vi "TempControl.vi"(0 "Param":sgl[](array[numeric])=[0.0, 0.0, 0.0, 0.0, 100.0, 10.0, 0.01, 0.005]) -> ()   [LabVIEW 2015]
uses:
  <vilib>/Instr/_visa.llb/VISA Configure Serial Port (Instr).vi
panel:
  out "error out 5":errorcluster
  in  "error in (no error) 5":errorcluster
  out "error out 4":errorcluster
  in  "error in (no error) 4":errorcluster
  out "error out 3":errorcluster
  in  "error in (no error) 3":errorcluster
  out "error out 2":errorcluster
  in  "error in (no error) 2":errorcluster
  in  "error in (no error)":errorcluster
  out "error out":errorcluster
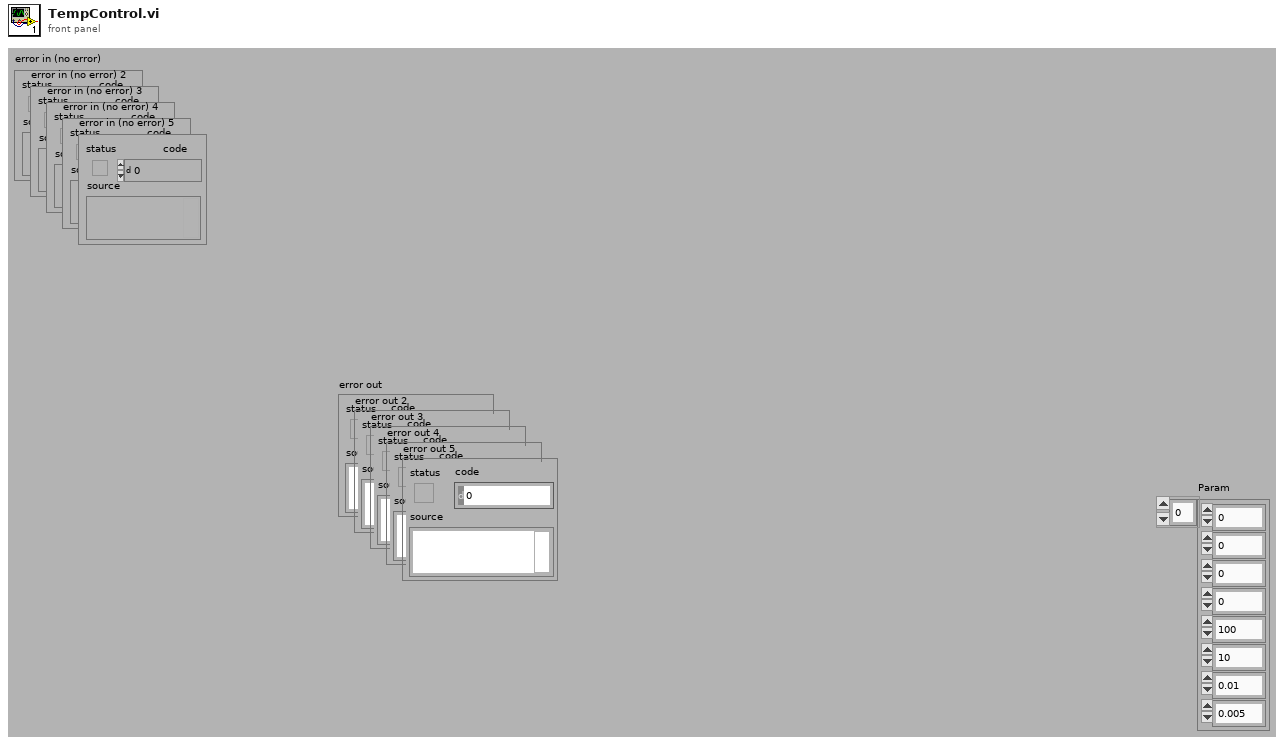
[diagram p1: front panel]
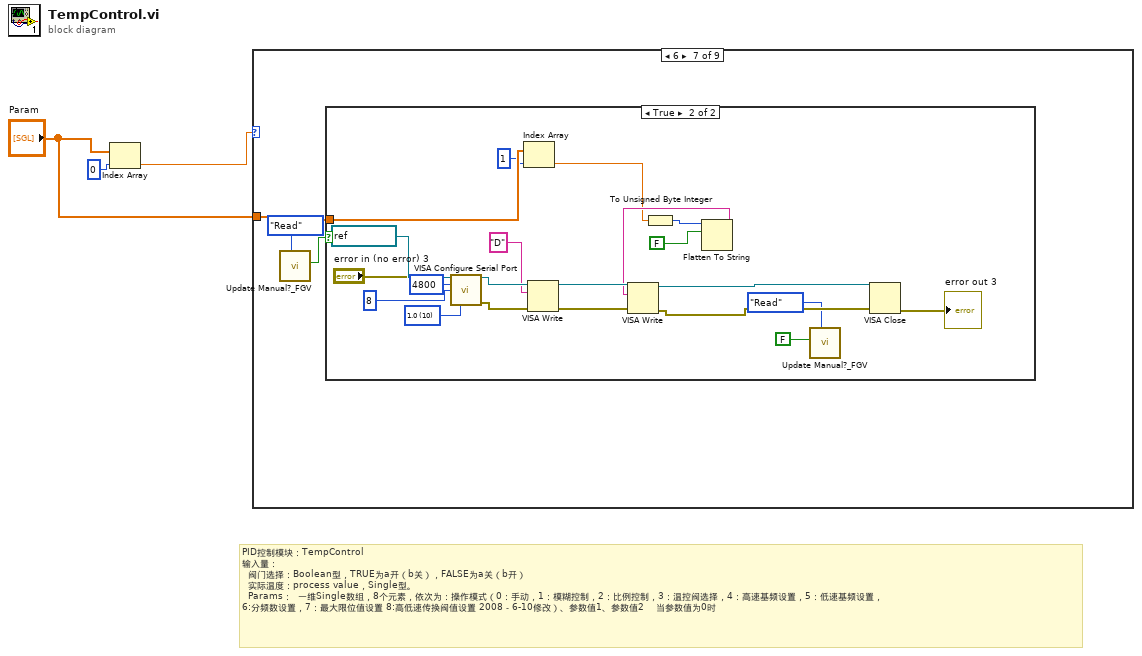
[diagram p0: block diagram]
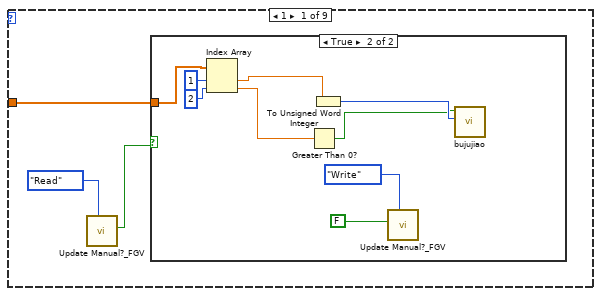
[diagram p2: hidden frame]
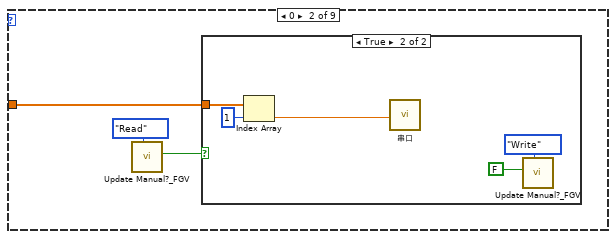
[diagram p4: hidden frame]
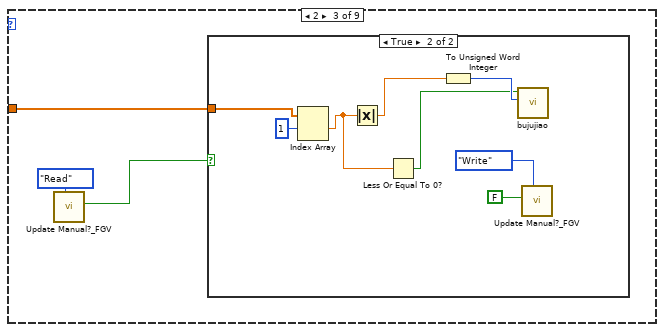
[diagram p6: hidden frame]
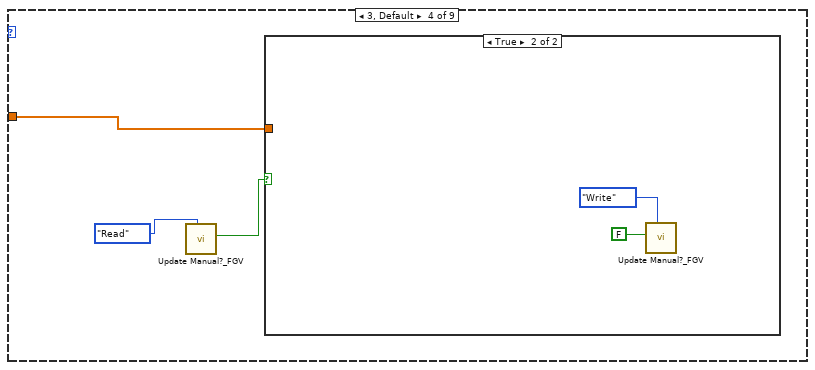
[diagram p8: hidden frame]
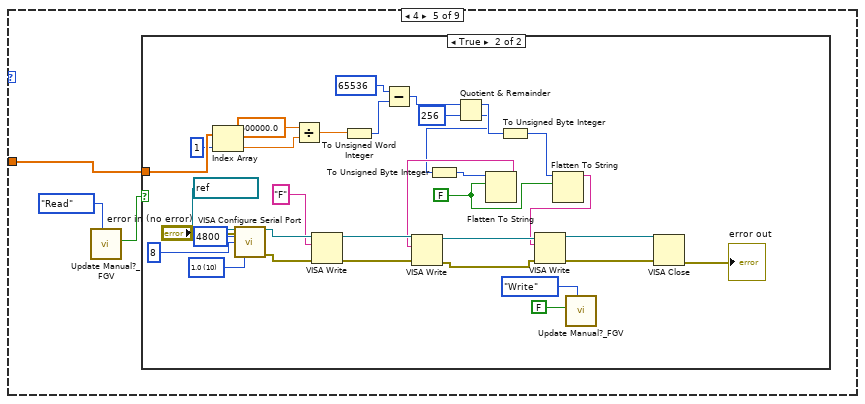
[diagram p10: hidden frame]
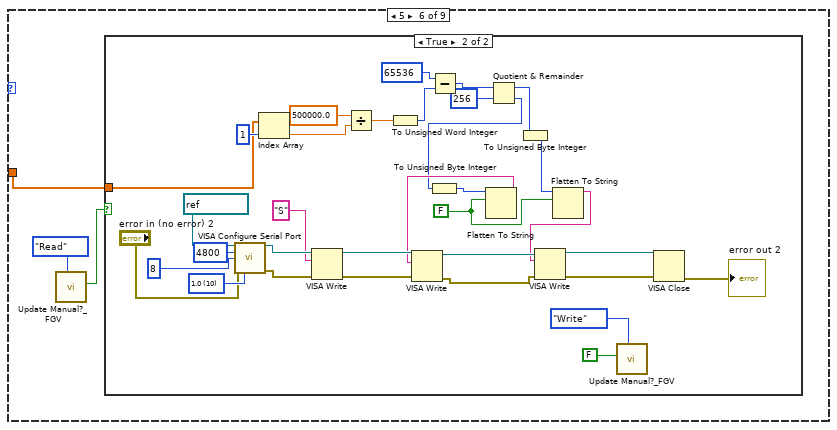
[diagram p12: hidden frame]
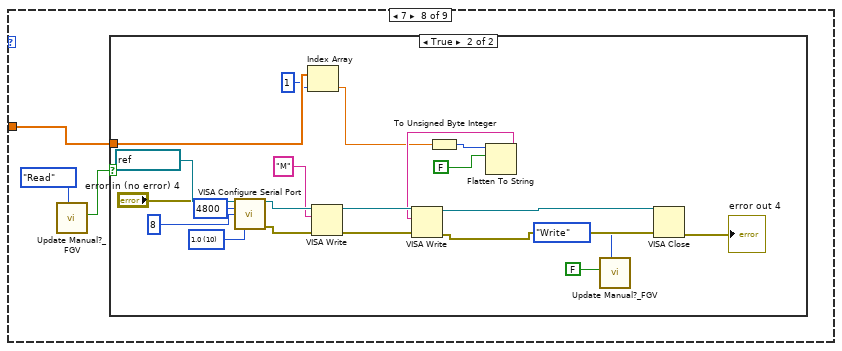
[diagram p15: hidden frame]
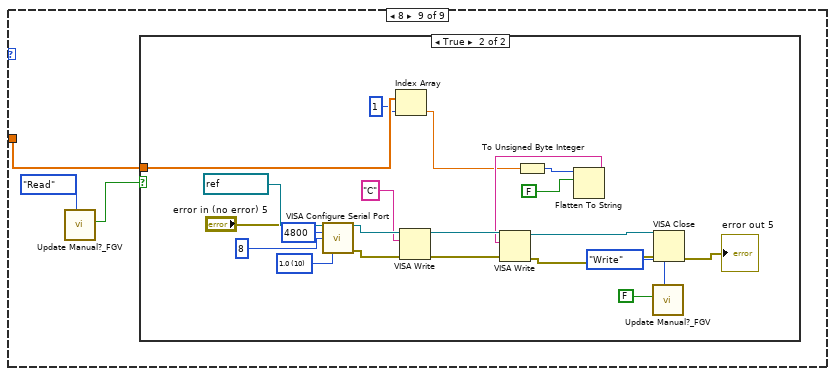
[diagram p17: hidden frame]
diagram:
  # "PID控制模块：TempControl\n输入量： \n \t阀门选择：Boolean型，TRUE为a开（b关），FALSE为a关（b开）\n \t实际温度：process value，Single型。\n \tParams：  一维Single数组，8个元素，依次为：操作模式（0：手动，1：模糊控制，2：比例控制，3：温控阀选择，4：高速基频设置，5：低速基频设置，\n6:分频数设置，7：最大限位值设置 8:高低速传换阀值设置 2008－6-10修改）、参数值1、参数值2    当参数值为0时"
  n1 = Index Array(array="Param", index=0) -> (element=w2:sgl)
  n2 = case shown="6" w2 {
    tunnel: "Param" -> [w6 w18 w26 w35 w42 w78 w114 w138 w162]
    frame 1 {
      n3 = call "Update Manual?_FGV.vi"("W/R"=enum16{"Write", "Read"}."Read") -> ("Update Manual Output?"=w4:bool)  [unwired: 10 in]
      n4 = case shown="True" w4 {
        tunnel: w6 -> [_ w15]
        frame False {
        }
        frame True {
          n5 = Index Array(array=w15, index #1=1 ("index"), index #2=2 ("index")) -> (element #1=w13:sgl, element #2=w10:sgl)
          n6 = Greater Than 0?(x=w10) -> (x > 0?=w9:bool)
          n7 = To Unsigned Word Integer(number=w13) -> (unsigned 16bit integer=w11:u16)
          n8 = call "Update Manual?_FGV.vi"("W/R"=enum16{"Write", "Read"}."Write", "Update Manual?"=FALSE) -> ()  [unwired: 9 in, 1 out]
          n9 = call "bujujiao.vi"("stepnum"=w11, "OK Button"=w9) -> ()  [unwired: 10 in]
        }
      }
    }
    frame 0 {
      n10 = call "Update Manual?_FGV.vi"("W/R"=enum16{"Write", "Read"}."Read") -> ("Update Manual Output?"=w17:bool)  [unwired: 10 in]
      n11 = case shown="True" w17 {
        tunnel: w18 -> [_ w23]
        frame False {
        }
        frame True {
          n12 = Index Array(array=w23, index=1) -> (element=w19:sgl)
          n13 = call "串口.vi"("电压值"=w19) -> ()  [unwired: 10 in, 1 out]
          n14 = call "Update Manual?_FGV.vi"("W/R"=enum16{"Write", "Read"}."Write", "Update Manual?"=FALSE) -> ()  [unwired: 9 in, 1 out]
        }
      }
    }
    frame 2 {
      n15 = call "Update Manual?_FGV.vi"("W/R"=enum16{"Write", "Read"}."Read") -> ("Update Manual Output?"=w24:bool)  [unwired: 10 in]
      n16 = case shown="True" w24 {
        tunnel: w26 -> [_ w34]
        frame False {
        }
        frame True {
          n17 = Index Array(array=w34, index #1=1 ("index")) -> (element #1=w27:sgl)  [unwired: 1 in, 1 out]
          n18 = Absolute Value(x=w27) -> (abs(x)=w30:sgl)
          n19 = Less Or Equal To 0?(x=w27) -> (x <= 0?=w31:bool)
          n20 = To Unsigned Word Integer(number=w30) -> (unsigned 16bit integer=w32:u16)
          n21 = call "bujujiao.vi"("stepnum"=w32, "OK Button"=w31) -> ()  [unwired: 10 in]
          n22 = call "Update Manual?_FGV.vi"("W/R"=enum16{"Write", "Read"}."Write", "Update Manual?"=FALSE) -> ()  [unwired: 9 in, 1 out]
        }
      }
    }
    frame 3, Default {
      n23 = call "Update Manual?_FGV.vi"("W/R"=enum16{"Write", "Read"}."Read") -> ("Update Manual Output?"=w37:bool)  [unwired: 10 in]
      n24 = case shown="True" w37 {
        tunnel: w35 -> [_ _]
        frame False {
        }
        frame True {
          n25 = call "Update Manual?_FGV.vi"("W/R"=enum16{"Write", "Read"}."Write", "Update Manual?"=FALSE) -> ()  [unwired: 9 in, 1 out]
        }
      }
    }
    frame 4 {
      n26 = call "Update Manual?_FGV.vi"("W/R"=enum16{"Write", "Read"}."Read") -> ("Update Manual Output?"=w41:bool)  [unwired: 10 in]
      n27 = case shown="True" w41 {
        tunnel: w42 -> [_ w55]
        frame False {
        }
        frame True {
          w65 = u16 10 items=["1.0"=10, "1.5"=15, "2.0"=20] ("stop bits (10: 1 bit)")
          w57 = FALSE ("prepend array or string size? (T)")
          n28 = Index Array(array=w55, index=1) -> (element=w51:sgl)
          n29 = call-poly "VISA Configure Serial Port"("VISA resource name"=refnum<visa-resource-name> "COM1", "baud rate (9600)"=u32 4800, "data bits (8)"=u16 8, "error in (no error)"="error in (no error)", "stop bits (10: 1 bit)"=w65) -> ("VISA resource name out"=w75:refnum<visa-resource-name>, "error out"=w71:errorcluster)  [unwired: 9 in]
          n30 = Divide(x=sgl 500000.0, y=w51) -> (x/y=w49:sgl)
          n31 = VISA Write(VISA resource name=w75, write buffer="F", error in (no error)=w71) -> (VISA resource name out=w68:refnum<visa-resource-name>, error out=w67:errorcluster)  [unwired: 1 out]
          n32 = To Unsigned Word Integer(number=w49) -> (unsigned 16bit integer=w52:u16)
          n33 = Subtract(x=65536, y=w52) -> (x-y=w48:i32)
          n34 = Quotient & Remainder(x=w48, y=256) -> (x-y*floor(x/y)=w46:i32, floor(x/y)=w45:i32)
          n35 = To Unsigned Byte Integer(number=w45) -> (unsigned 8bit integer=w70:u8)
          n36 = Flatten To String(anything=w70, prepend array or string size? (T)=w57) -> (data string=w66:string)  [unwired: 2 in, 2 out]
          n37 = VISA Write(VISA resource name=w68, write buffer=w66, error in (no error)=w67) -> (VISA resource name out=w62:refnum<visa-resource-name>, error out=w59:errorcluster)  [unwired: 1 out]
          n38 = To Unsigned Byte Integer(number=w46) -> (unsigned 8bit integer=w58:u8)
          n39 = Flatten To String(anything=w58, prepend array or string size? (T)=w57) -> (data string=w56:string)  [unwired: 2 in, 2 out]
          n40 = VISA Write(VISA resource name=w62, write buffer=w56, error in (no error)=w59) -> (VISA resource name out=w61:refnum<visa-resource-name>, error out=w60:errorcluster)  [unwired: 1 out]
          n41 = call "Update Manual?_FGV.vi"("W/R"=enum16{"Write", "Read"}."Write", "Update Manual?"=FALSE) -> ()  [unwired: 9 in, 1 out]
          n42 = VISA Close(VISA resource name=w61, error in (no error)=w60) -> (error out=→"error out":errorcluster)
        }
      }
    }
    frame 5 {
      n43 = call "Update Manual?_FGV.vi"("W/R"=enum16{"Write", "Read"}."Read") -> ("Update Manual Output?"=w77:bool)  [unwired: 10 in]
      n44 = case shown="True" w77 {
        tunnel: w78 -> [_ w86]
        frame False {
        }
        frame True {
          w101 = u16 10 items=["1.0"=10, "1.5"=15, "2.0"=20] ("stop bits (10: 1 bit)")
          w94 = FALSE ("prepend array or string size? (T)")
          n45 = call-poly "VISA Configure Serial Port"("VISA resource name"=refnum<visa-resource-name> "COM1", "baud rate (9600)"=u32 4800, "data bits (8)"=u16 8, "error in (no error)"="error in (no error) 2", "stop bits (10: 1 bit)"=w101) -> ("VISA resource name out"=w111:refnum<visa-resource-name>, "error out"=w107:errorcluster)  [unwired: 9 in]
          n46 = Index Array(array=w86, index=1) -> (element=w91:sgl)
          n47 = VISA Write(VISA resource name=w111, write buffer="S", error in (no error)=w107) -> (VISA resource name out=w104:refnum<visa-resource-name>, error out=w103:errorcluster)  [unwired: 1 out]
          n48 = Divide(x=sgl 500000.0, y=w91) -> (x/y=w89:sgl)
          n49 = To Unsigned Word Integer(number=w89) -> (unsigned 16bit integer=w87:u16)
          n50 = Subtract(x=65536, y=w87) -> (x-y=w85:i32)
          n51 = Quotient & Remainder(x=w85, y=256) -> (x-y*floor(x/y)=w82:i32, floor(x/y)=w83:i32)
          n52 = To Unsigned Byte Integer(number=w83) -> (unsigned 8bit integer=w106:u8)
          n53 = Flatten To String(anything=w106, prepend array or string size? (T)=w94) -> (data string=w102:string)  [unwired: 2 in, 2 out]
          n54 = VISA Write(VISA resource name=w104, write buffer=w102, error in (no error)=w103) -> (VISA resource name out=w98:refnum<visa-resource-name>, error out=w95:errorcluster)  [unwired: 1 out]
          n55 = To Unsigned Byte Integer(number=w82) -> (unsigned 8bit integer=w81:u8)
          n56 = Flatten To String(anything=w81, prepend array or string size? (T)=w94) -> (data string=w93:string)  [unwired: 2 in, 2 out]
          n57 = VISA Write(VISA resource name=w98, write buffer=w93, error in (no error)=w95) -> (VISA resource name out=w97:refnum<visa-resource-name>, error out=w96:errorcluster)  [unwired: 1 out]
          n58 = call "Update Manual?_FGV.vi"("W/R"=enum16{"Write", "Read"}."Write", "Update Manual?"=FALSE) -> ()  [unwired: 9 in, 1 out]
          n59 = VISA Close(VISA resource name=w97, error in (no error)=w96) -> (error out=→"error out 2":errorcluster)
        }
      }
    }
    frame 6 {
      n60 = call "Update Manual?_FGV.vi"("W/R"=enum16{"Write", "Read"}."Read") -> ("Update Manual Output?"=w113:bool)  [unwired: 10 in]
      n61 = case shown="True" w113 {
        tunnel: w114 -> [_ w122]
        frame False {
        }
        frame True {
          w125 = u16 10 items=["1.0"=10, "1.5"=15, "2.0"=20] ("stop bits (10: 1 bit)")
          n62 = call-poly "VISA Configure Serial Port"("VISA resource name"=refnum<visa-resource-name> "COM1", "baud rate (9600)"=u32 4800, "data bits (8)"=u16 8, "error in (no error)"="error in (no error) 3", "stop bits (10: 1 bit)"=w125) -> ("VISA resource name out"=w135:refnum<visa-resource-name>, "error out"=w131:errorcluster)  [unwired: 9 in]
          n63 = Index Array(array=w122, index=1) -> (element=w117:sgl)
          n64 = VISA Write(VISA resource name=w135, write buffer="D", error in (no error)=w131) -> (VISA resource name out=w128:refnum<visa-resource-name>, error out=w127:errorcluster)  [unwired: 1 out]
          n65 = To Unsigned Byte Integer(number=w117) -> (unsigned 8bit integer=w130:u8)
          n66 = Flatten To String(anything=w130, prepend array or string size? (T)=FALSE) -> (data string=w126:string)  [unwired: 2 in, 2 out]
          n67 = VISA Write(VISA resource name=w128, write buffer=w126, error in (no error)=w127) -> (VISA resource name out=w119:refnum<visa-resource-name>, error out=w118:errorcluster)  [unwired: 1 out]
          n68 = call "Update Manual?_FGV.vi"("W/R"=enum16{"Write", "Read"}."Read", "Update Manual?"=FALSE) -> ()  [unwired: 9 in, 1 out]
          n69 = VISA Close(VISA resource name=w119, error in (no error)=w118) -> (error out=→"error out 3":errorcluster)
        }
      }
    }
    frame 7 {
      n70 = call "Update Manual?_FGV.vi"("W/R"=enum16{"Write", "Read"}."Read") -> ("Update Manual Output?"=w136:bool)  [unwired: 10 in]
      n71 = case shown="True" w136 {
        tunnel: w138 -> [_ w146]
        frame False {
        }
        frame True {
          w149 = u16 10 items=["1.0"=10, "1.5"=15, "2.0"=20] ("stop bits (10: 1 bit)")
          n72 = call-poly "VISA Configure Serial Port"("VISA resource name"=refnum<visa-resource-name> "COM1", "baud rate (9600)"=u32 4800, "data bits (8)"=u16 8, "error in (no error)"="error in (no error) 4", "stop bits (10: 1 bit)"=w149) -> ("VISA resource name out"=w159:refnum<visa-resource-name>, "error out"=w155:errorcluster)  [unwired: 9 in]
          n73 = Index Array(array=w146, index=1) -> (element=w144:sgl)
          n74 = VISA Write(VISA resource name=w159, write buffer="M", error in (no error)=w155) -> (VISA resource name out=w152:refnum<visa-resource-name>, error out=w151:errorcluster)  [unwired: 1 out]
          n75 = To Unsigned Byte Integer(number=w144) -> (unsigned 8bit integer=w154:u8)
          n76 = Flatten To String(anything=w154, prepend array or string size? (T)=FALSE) -> (data string=w150:string)  [unwired: 2 in, 2 out]
          n77 = VISA Write(VISA resource name=w152, write buffer=w150, error in (no error)=w151) -> (VISA resource name out=w142:refnum<visa-resource-name>, error out=w141:errorcluster)  [unwired: 1 out]
          n78 = call "Update Manual?_FGV.vi"("W/R"=enum16{"Write", "Read"}."Write", "Update Manual?"=FALSE) -> ()  [unwired: 9 in, 1 out]
          n79 = VISA Close(VISA resource name=w142, error in (no error)=w141) -> (error out=→"error out 4":errorcluster)
        }
      }
    }
    frame 8 {
      n80 = call "Update Manual?_FGV.vi"("W/R"=enum16{"Write", "Read"}."Read") -> ("Update Manual Output?"=w160:bool)  [unwired: 10 in]
      n81 = case shown="True" w160 {
        tunnel: w162 -> [_ w170]
        frame False {
        }
        frame True {
          w173 = u16 10 items=["1.0"=10, "1.5"=15, "2.0"=20] ("stop bits (10: 1 bit)")
          n82 = call-poly "VISA Configure Serial Port"("VISA resource name"=refnum<visa-resource-name> "COM1", "baud rate (9600)"=u32 4800, "data bits (8)"=u16 8, "error in (no error)"="error in (no error) 5", "stop bits (10: 1 bit)"=w173) -> ("VISA resource name out"=w183:refnum<visa-resource-name>, "error out"=w179:errorcluster)  [unwired: 9 in]
          n83 = Index Array(array=w170, index=1) -> (element=w168:sgl)
          n84 = VISA Write(VISA resource name=w183, write buffer="C", error in (no error)=w179) -> (VISA resource name out=w176:refnum<visa-resource-name>, error out=w175:errorcluster)  [unwired: 1 out]
          n85 = To Unsigned Byte Integer(number=w168) -> (unsigned 8bit integer=w178:u8)
          n86 = Flatten To String(anything=w178, prepend array or string size? (T)=FALSE) -> (data string=w174:string)  [unwired: 2 in, 2 out]
          n87 = VISA Write(VISA resource name=w176, write buffer=w174, error in (no error)=w175) -> (VISA resource name out=w166:refnum<visa-resource-name>, error out=w165:errorcluster)  [unwired: 1 out]
          n88 = call "Update Manual?_FGV.vi"("W/R"=enum16{"Write", "Read"}."Write", "Update Manual?"=FALSE) -> ()  [unwired: 9 in, 1 out]
          n89 = VISA Close(VISA resource name=w166, error in (no error)=w165) -> (error out=→"error out 5":errorcluster)
        }
      }
    }
  }
